vi "Pigeon2Set.vi"   [LabVIEW 2023]
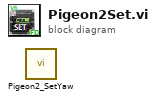
[diagram p0: block diagram]
diagram:
  n1 = call <vilib>:"Pigeon2_SetYaw.vi"() -> ()  [unwired: 11 in, 1 out]
